vi "Write SS with head and dialog prompt.vi"(0 "Header String":string=" ", 2 "file path":path, 7 "Data to Write":dbl[][](array[numeric])=[[0.0, 0.0], [0.0, 2.0]] format="%.2f", 11 "Transpose Data?":bool, 13 "use int dialog (default=T)":bool=TRUE) -> ()   [LabVIEW 2019]
doc: "This vi writes a 2D spreadsheet to file and includes a text header. It is meant to work specifically with Read SS with Header.vi\n\nIt uses the default prompt for a filename.\n\nThe parser string is [CR, CR, \"<data below>\", CR, CR].\n\nThe error handling is embedded.\n\nPaul K Dixon\nP3600\nCSUSB Physics"
uses:
  <vilib>/Utility/file.llb/Write Delimited Spreadsheet (DBL).vi
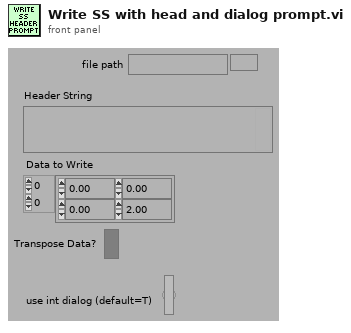
[diagram p1: front panel]
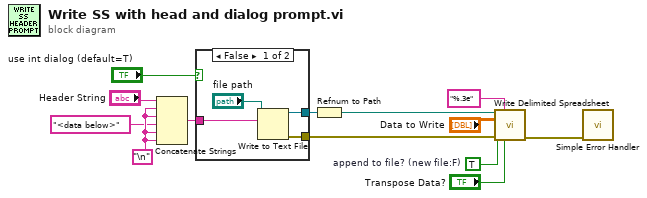
[diagram p0: block diagram]
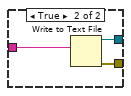
[diagram p2: hidden frame]
diagram:
  w7 = TRUE  # append to file? (new file:F)
  w9 = "\n"
  n1 = Concatenate Strings("Header String", w9, w9, "<data below>", w9, w9) -> (w6:string)
  n2 = case shown="False" "use int dialog (default=T)" {
    tunnel: w6 -> [w17 w20]
    tunnel: [w16 w19] -> w5
    tunnel: [w14 w18] -> w3
    frame False {
      n3 = Write to Text File(file (use dialog)="file path", text=w17) -> (refnum out=w16:refnum<file>, error out=w14:errorcluster)  [unwired: 2 in, 1 out]
    }
    frame True {
      n4 = Write to Text File(text=w20) -> (refnum out=w19:refnum<file>, error out=w18:errorcluster)  [unwired: 3 in, 1 out]
    }
  }
  n5 = Refnum to Path(1:w5) -> (0:w4:path)
  n6 = call-poly <vilib>:"Write Delimited Spreadsheet.vi"("file path (dialog if empty)"=w4, "format (%.3f)"="%.3e", "2D data"="Data to Write", "append to file? (new file:F)"=w7, "error in (no error)"=w3, "transpose? (no:F)"="Transpose Data?") -> ("error out"=w2:errorcluster)  [unwired: 8 in, 1 out]
  n7 = call <vilib>:"Simple Error Handler.vi"("error in (no error)"=w2) -> ()  [unwired: 4 in, 5 out]
